vi "Open Sensors.vi"   [LabVIEW 2014]
uses:
  <vilib>/Rock Robotics/SystemInterfaces/AI/FPGA_AIGyroChannel.ctl
  Robot Global Data.vi
  <vilib>/Rock Robotics/WPI/Switch/WPI_SwitchOpenLimit.vi
  <vilib>/Rock Robotics/WPI/Counter/WPI_CounterDigitalInputToDigitalSource.vi
types:
  T1 = typedef "FPGA_AIGyroChannel.ctl" = enum8{"AI 0", "AI 1", "Invalid"}
  T2 = typedef "FPGA_DIOChannel.ctl" = enum8{"DIO 0", "DIO 1", "DIO 2", "DIO 3", "DIO 4", "DIO 5", "DIO 6", "DIO 7", "DIO 8", "DIO 9", "DIO MXP 0", "DIO MXP 1", "DIO MXP 2", "DIO MXP 3", "DIO MXP 4", "DIO MXP 5", "DIO MXP 6", "DIO MXP 7", "DIO MXP 8", "DIO MXP 9", "DIO MXP 10", "DIO MXP 11", "DIO MXP 12", "DIO MXP 13", "DIO MXP 14", "DIO MXP 15", "Invalid"}
  T3 = cluster{"Lift Motors":cluster{"Left Lift":dbl, "Right Lift":dbl}, "Sensors":cluster{"Limit Switches":cluster{"Top IR":T2, "Bottom IR":T2, "Lift Safety":T2, "Lower IR":T2, "Middle IR":T2, "Upper IR":T2}, "Encoders":cluster{"Lift Encoder A Pin":T2, "Lift Encoder B Pin":T2}}, "Solenoids":cluster{"Upper Clamp FWD":dbl, "Lower Clamp FWD":dbl, "Brake BCK":dbl, "Upper Clamp BCK":dbl, "Lower Clamp BCK":dbl, "Upper Clamp PModule":dbl, "Lower Clamp PModule":dbl, "Brake PModule":dbl, "Brake FWD":dbl}, "Drive Motors":cluster{"Rear Left Motor":dbl, "Rear Right Motor":dbl, "Front Left Motor":dbl, "Front Right Motor":dbl}, "Compressor":dbl}
  T4 = typedef "WPI_SwitchDevRef.ctl" = cluster{"DevStatus":errorcluster, "DIO Channel":T2, "Controller":T5, "CntIndex":T6, "Normally Closed":bool}
  T5 = typedef "FPGA_TypedefDigitalModule.ctl" = enum16{"Controller 1"}
  T6 = typedef "FPGA_CounterCtrSystemIndex.ctl" = enum8{"Ctr 0", "Ctr 1", "Ctr 2", "Ctr 3", "Ctr 4", "Ctr 5", "Ctr 6", "Ctr 7", "Invalid"}
  T7 = typedef "WPI_DigitalInputDevRef.ctl" = cluster{"DevStatus":errorcluster, "DIO Channel":T2, "Controller":T5}
  T8 = typedef "FPGA_CounterEncoderSourceConvertionLVSourceType.ctl" = cluster{"DevStatus":errorcluster, "AnalogTriggerMode?":bool, "DigitalMode":cluster{"Controller":T5, "DIO Channel":T9}, "AnalogTriggerMode":cluster{"AnalogTriggerIndex":T10, "OutputType":T11}}
  T9 = typedef "FPGA_DIODigitalSourceChannel.ctl" = enum8{"DIO 0", "DIO 1", "DIO 2", "DIO 3", "DIO 4", "DIO 5", "DIO 6", "DIO 7", "DIO 8", "DIO 9", "DIO MXP 0", "DIO MXP 1", "DIO MXP 2", "DIO MXP 3", "DIO MXP 4", "DIO MXP 5", "DIO MXP 6", "DIO MXP 7", "DIO MXP 8", "DIO MXP 9", "DIO MXP 10", "DIO MXP 11", "DIO MXP 12", "DIO MXP 13", "DIO MXP 14", "DIO MXP 15", "Disabled"}
  T10 = typedef "FPGA_AnalogTriggerIndex.ctl" = enum8{"Trig 0", "Trig 1", "Trig 2", "Trig 3", "Trig 4", "Trig 5", "Trig 6", "Trig 7", "Invalid"}
  T11 = typedef "FPGA_AnalogTriggerOutType.ctl" = enum16{"InWindow", "TriggerState", "Rising", "Falling"}
  T12 = typedef "WPI_EncoderDevRef.ctl" = cluster{"DevStatus":errorcluster, "EncoderIndex":T13, "CounterIndex":T6, "DistancePerCount":dbl, "Decoding Type":T14}
  T13 = typedef "FPGA_EncoderIdx.ctl" = enum8{"Enc 0", "Enc 1", "Enc 2", "Enc 3", "Enc 4", "Enc 5", "Enc 6", "Enc 7", "Invalid"}
  T14 = typedef "WPI_EncoderType.ctl" = enum16{"1x", "2x", "4x"}
  T15 = typedef "WPI_GyroDevRef.ctl" = cluster{"DevStatus":errorcluster, "Analog Module":T16, "Analog Channel":T17, "Offset":dbl, "Gain (VoltsPerDegree/Second)":dbl}
  T16 = typedef "FPGA_TypedefAnalogModule.ctl" = enum16{"Controller 1"}
  T17 = typedef "FPGA_AIChannel.ctl" = enum8{"AI 0", "AI 1", "AI 2", "AI 3", "AI MXP 0", "AI MXP 1", "AI MXP 2", "AI MXP 3", "Invalid"}
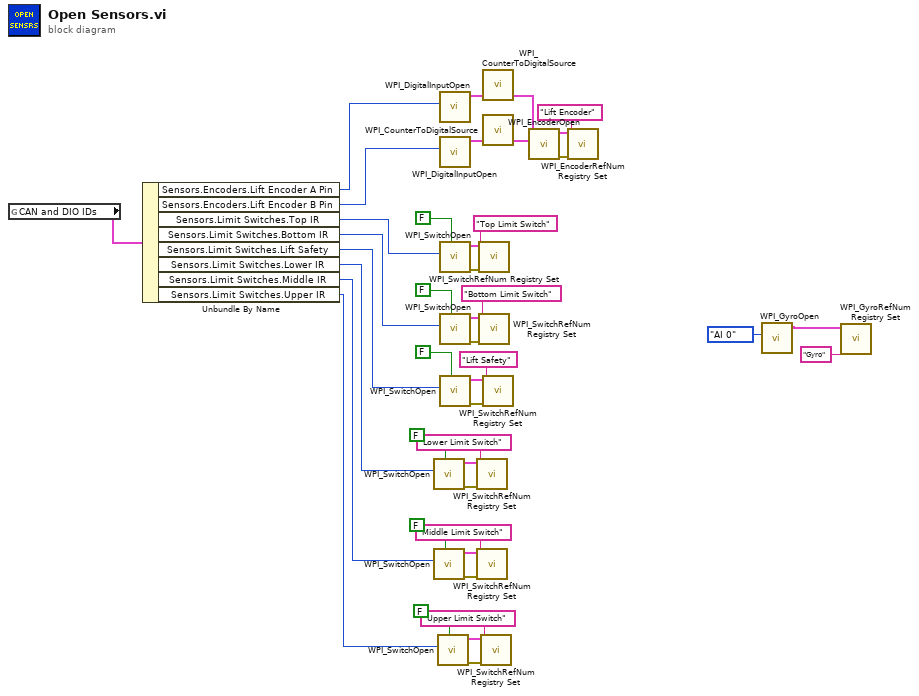
[diagram p0: block diagram]
diagram:
  n1 = global read "Robot Global Data.vi" "CAN and DIO IDs"() -> (w39:T3)
  n2 = Unbundle By Name(w39) -> ("Sensors.Encoders.Lift Encoder A Pin"=w38:T2, "Sensors.Encoders.Lift Encoder B Pin"=w37:T2, "Sensors.Limit Switches.Top IR"=w25:T2, "Sensors.Limit Switches.Bottom IR"=w24:T2, "Sensors.Limit Switches.Lift Safety"=w22:T2, "Sensors.Limit Switches.Lower IR"=w11:T2, "Sensors.Limit Switches.Middle IR"=w2:T2, "Sensors.Limit Switches.Upper IR"=w1:T2)
  n3 = call-poly <vilib>:"WPI_SwitchOpen.vi"("Normally Closed"=FALSE, "DIO Channel"=w11) -> ("error out"=w13:errorcluster, "SwitchDevRef"=w14:T4)  [unwired: 8 in]
  n4 = call-poly <vilib>:"WPI_SwitchOpen.vi"("Normally Closed"=FALSE, "DIO Channel"=w2) -> ("error out"=w9:errorcluster, "SwitchDevRef"=w8:T4)  [unwired: 8 in]
  n5 = call-poly <vilib>:"WPI_SwitchOpen.vi"("Normally Closed"=FALSE, "DIO Channel"=w1) -> ("error out"=w4:errorcluster, "SwitchDevRef"=w5:T4)  [unwired: 8 in]
  n6 = call <vilib>:"WPI_DigitalInputOpen.vi"("DIO Channel"=w38) -> ("DigitalInputDevRef"=w41:T7)  [unwired: 2 in, 8 out]
  n7 = call <vilib>:"WPI_DigitalInputOpen.vi"("DIO Channel"=w37) -> ("DigitalInputDevRef"=w42:T7)  [unwired: 2 in, 8 out]
  n8 = call-poly <vilib>:"WPI_SwitchOpen.vi"("Normally Closed"=FALSE, "DIO Channel"=w25) -> ("error out"=w29:errorcluster, "SwitchDevRef"=w28:T4)  [unwired: 8 in]
  n9 = call-poly <vilib>:"WPI_SwitchOpen.vi"("Normally Closed"=FALSE, "DIO Channel"=w24) -> ("error out"=w31:errorcluster, "SwitchDevRef"=w30:T4)  [unwired: 8 in]
  n10 = call-poly <vilib>:"WPI_SwitchOpen.vi"("Normally Closed"=FALSE, "DIO Channel"=w22) -> ("error out"=w21:errorcluster, "SwitchDevRef"=w20:T4)  [unwired: 8 in]
  n11 = call <vilib>:"WPI_SwitchRefNum Registry Set.vi"("error in (no error)"=w13, "refnum name"="Lower Limit Switch", "SwitchDevRef"=w14) -> ()  [unwired: 7 in, 2 out]
  n12 = call <vilib>:"WPI_SwitchRefNum Registry Set.vi"("error in (no error)"=w9, "refnum name"="Middle Limit Switch", "SwitchDevRef"=w8) -> ()  [unwired: 7 in, 2 out]
  n13 = call <vilib>:"WPI_SwitchRefNum Registry Set.vi"("error in (no error)"=w29, "refnum name"="Top Limit Switch", "SwitchDevRef"=w28) -> ()  [unwired: 7 in, 2 out]
  n14 = call <vilib>:"WPI_SwitchRefNum Registry Set.vi"("error in (no error)"=w31, "refnum name"="Bottom Limit Switch", "SwitchDevRef"=w30) -> ()  [unwired: 7 in, 2 out]
  n15 = call <vilib>:"WPI_SwitchRefNum Registry Set.vi"("error in (no error)"=w4, "refnum name"="Upper Limit Switch", "SwitchDevRef"=w5) -> ()  [unwired: 7 in, 2 out]
  n16 = call-poly <vilib>:"WPI_CounterToDigitalSource.vi"("DigitalInputDevRef"=w41) -> ("Digital Source"=w40:T8)  [unwired: 6 out]
  n17 = call-poly <vilib>:"WPI_CounterToDigitalSource.vi"("DigitalInputDevRef"=w42) -> ("Digital Source"=w43:T8)  [unwired: 6 out]
  n18 = call <vilib>:"WPI_SwitchRefNum Registry Set.vi"("error in (no error)"=w21, "refnum name"="Lift Safety", "SwitchDevRef"=w20) -> ()  [unwired: 7 in, 2 out]
  n19 = call <vilib>:"WPI_EncoderOpen.vi"("BSource"=w43, "ASource"=w40) -> ("error out"=w36:errorcluster, "EncoderDevRef"=w35:T12)  [unwired: 6 in, 2 out]
  n20 = call <vilib>:"WPI_EncoderRefNum Registry Set.vi"("error in (no error)"=w36, "refnum name"="Lift Encoder", "EncoderDevRef"=w35) -> ()  [unwired: 7 in, 2 out]
  n21 = call <vilib>:"WPI_GyroOpen.vi"("Analog Channel"=FPGA_AIGyroChannel."AI 0") -> ("GyroDevRef"=w17:T15)  [unwired: 8 in, 2 out]
  n22 = call <vilib>:"WPI_GyroRefNum Registry Set.vi"("refnum name"="Gyro", "GyroDevRef"=w17) -> ()  [unwired: 8 in, 2 out]
